vi "Release.vi"(8 "error in (no error)":errorcluster, 11 "Mapped Buffer":refnum<data-value>) -> (0 "error out":errorcluster, 3 "Buffer":refnum<class "Buffer.lvclass">)   [LabVIEW 2020, in "Buffer Byte-Stream Access.lvclass"]
uses:
  Buffer Byte-Stream Access.lvclass
  Buffer/Buffer.lvclass
  Buffer Byte-Stream Access.lvclass/Buffer Byte-Stream Access.ctl
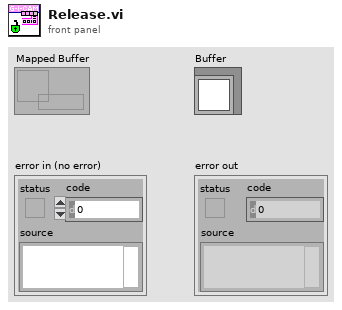
[diagram p1: front panel]
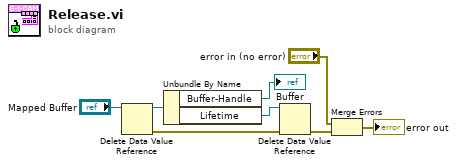
[diagram p0: block diagram]
diagram:
  n1 = Delete Data Value Reference(data value reference="Mapped Buffer") -> (data value=w7:refnum<class "Buffer Byte-Stream Access.lvclass">, error out=w5:errorcluster)  [unwired: 1 in]
  n2 = Unbundle By Name(w7) -> ("Buffer-Handle"=→"Buffer":refnum<class "Buffer.lvclass">, "Lifetime"=w6:refnum<data-value>)
  n3 = Delete Data Value Reference(data value reference=w6, error in=w5) -> (error out=w3:errorcluster)  [unwired: 1 out]
  n4 = Merge Errors("error in (no error)", w3) -> (→"error out":errorcluster)
